vi "Sort Array by Column.vi"(8 "Column to Sort":i32, 9 "Reverse Direction?":bool=TRUE, 11 "Unsorted Array":string[][](array[string])) -> (3 "Sorted Array":string[][](array[string]))   [LabVIEW 2017, in "Message Log.lvclass"]
uses:
  Message Log.lvclass
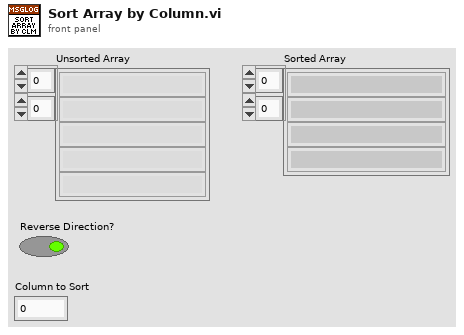
[diagram p1: front panel]
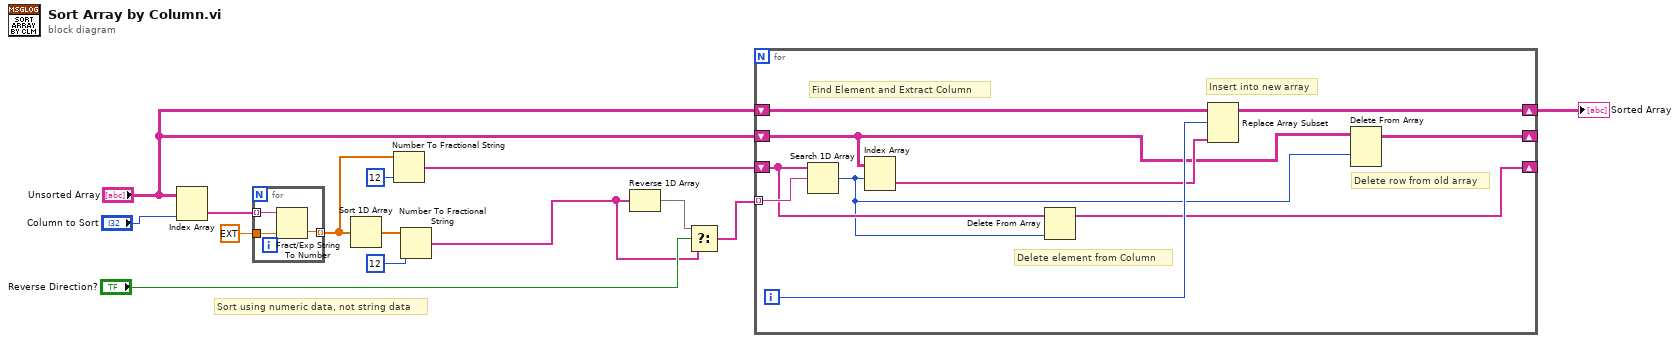
[diagram p0: block diagram]
diagram:
  # "Sort using numeric data, not string data"
  n1 = Index Array(array="Unsorted Array", index (col)="Column to Sort") -> (element=w7:string[])  [unwired: 1 in]
  n2 = for {
    tunnel: w7 -> [w17] mode=indexing
    tunnel: [w16] -> w3 mode=indexing
    tunnel: ext 0.0 -> [w15]
    n3 = Fract/Exp String To Number(string=w17, default (0 dbl)=w15) -> (number=w16:ext)  [unwired: 2 in, 1 out]
  }
  n4 = Sort 1D Array(array=w3) -> (sorted array=w8:ext[])
  n5 = Number To Fractional String(number=w3, precision (6)=i16 12) -> (F-format string=w6:string[])  [unwired: 2 in]
  n6 = Number To Fractional String(number=w8, precision (6)=i16 12) -> (F-format string=w5:string[])  [unwired: 2 in]
  n7 = Reverse 1D Array(array=w5) -> (reversed array=w11:string[])
  n8 = Select(t=w11, s="Reverse Direction?", f=w5) -> (s? t:f=w10:string[])
  n9 = for {
    tunnel: w10 -> [w27] mode=indexing
    shift-right: [w26] -> w12
    shift-left: "Unsorted Array" -> [w25]
    shift-right: [w21] -> _
    shift-left: w6 -> [w22]
    shift-right: [w20] -> _
    shift-left: "Unsorted Array" -> [w19]
    i -> [w24]
    # "Find Element and Extract Column"
    # "Delete element from Column"
    # "Delete row from old array"
    # "Insert into new array"
    n10 = Search 1D Array(1D array=w22, element=w27) -> (index of element=w18:i32)  [unwired: 1 in]
    n11 = Index Array(array=w19, index (row)=w18) -> (element=w23:string[])  [unwired: 1 in]
    n12 = Delete From Array(array=w22, index=w18) -> (array with subset deleted=w21:string[])  [unwired: 1 in, 1 out]
    n13 = Replace Array Subset(array=w25, new element=w23, index (row)=w24) -> (w26:string[][])  [unwired: 1 in]
    n14 = Delete From Array(array=w19, index (row)=w18) -> (array with subset deleted=w20:string[][])  [unwired: 2 in, 1 out]
  }
  "Sorted Array" <- w12
